vi "Save File DOE Parse Program Groups.vi"(4 "Headers":string[](array[string]), 9 "Search Name":string, 10 "Program Names":string[](array[string]), 11 "Model Information":string[][](array[string])) -> (3 "Parsed Program List":string[][](array[string]))   [LabVIEW 2016, in "File Setup.lvlib"]
uses:
  File Setup.lvlib
panel:
  in  "Header Search":string="Platform"
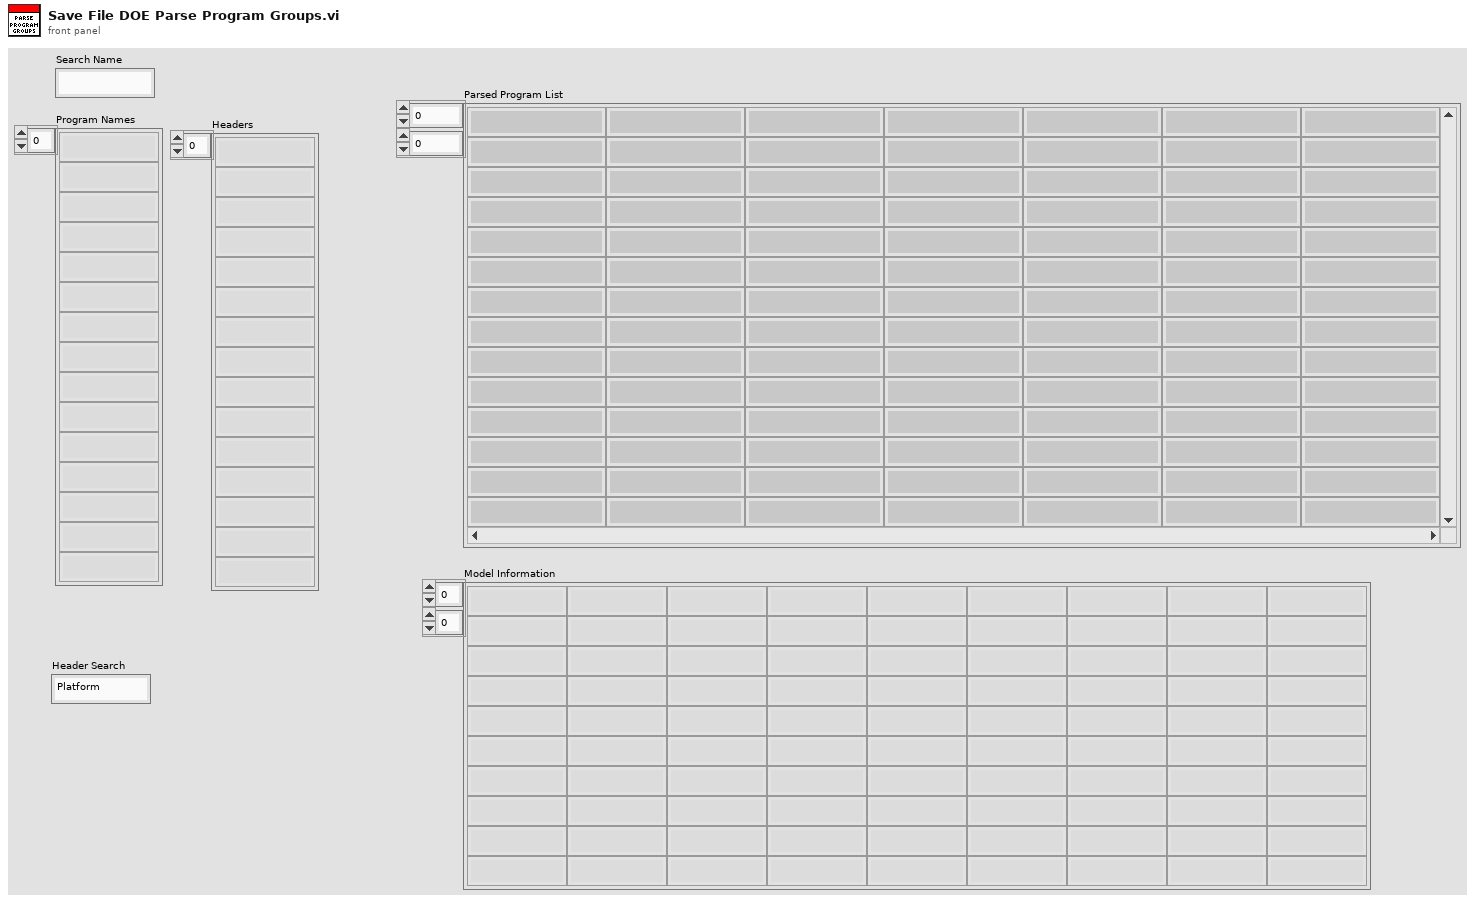
[diagram p1: front panel]
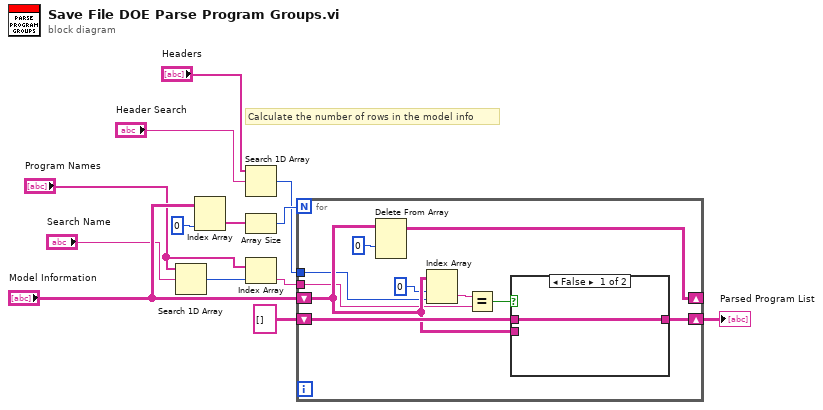
[diagram p0: block diagram]
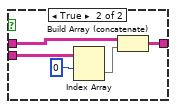
[diagram p2: hidden frame]
diagram:
  # "Calculate the number of rows in the model info"
  n1 = Search 1D Array(1D array="Program Names", element="Search Name") -> (index of element=w6:i32)  [unwired: 1 in]
  n2 = Index Array(array="Model Information", index (col)=0 ("disabled index (col)")) -> (element=w8:string[])  [unwired: 1 in]
  n3 = Search 1D Array(1D array="Headers", element="Header Search") -> (index of element=w1:i32)  [unwired: 1 in]
  n4 = Array Size(array=w8) -> (size(s)=w9:i32)
  n5 = Index Array(array="Program Names", index=w6) -> (element=w12:string)
  n6 = for {
    N: w9 -> [_]
    shift-right: [w22] -> w11
    shift-left: string[][] [] -> [w23]
    tunnel: w12 -> [w18]
    shift-right: [w20] -> _
    shift-left: "Model Information" -> [w21]
    tunnel: w1 -> [w14]
    n7 = Delete From Array(array=w21, index (row)=0) -> (array with subset deleted=w20:string[][])  [unwired: 2 in, 1 out]
    n8 = Index Array(array=w21, index (row)=0 ("disabled index (row)"), index (col)=w14) -> (element=w17:string)
    n9 = Equal?(x=w17, y=w18) -> (x = y?=w15:bool)
    n10 = case shown="False" w15 {
      tunnel: w21 -> [_ w29]
      tunnel: w23 -> [w24 w28]
      tunnel: [w24 w26] -> w22
      frame False {
      }
      frame True {
        n11 = Index Array(array=w29, index (row)=0) -> (element=w27:string[])  [unwired: 1 in]
        n12 = Build Array (concatenate)(w28, w27) -> (w26:string[][])
      }
    }
  }
  "Parsed Program List" <- w11
